vi "5. import Config.ini with include section.vi"() -> (3 "RS232_Device Config":T1={"Resource"="com5", "baud rate"=115200, "data bits"=8, "parity"=enum."Odd", "stop bits"=10})   [LabVIEW 2017]
doc: "## Referencing Configuration Files with [__include] (5. import Config.ini with include section.vi)\n\n### Overview\n\nThis example demonstrates CSM INI Variable Support API for referencing configuration files. You can use the reference configuration file feature to implement a distributed configuration file system.\n\n### Introduction\n\nIn configuration files loaded by CSM INI Variable Support API, if a [__include] section is present, the specified configuration files will be automatically referenced.\n\n**Notes:**\n\n- Relative paths are resolved relative to the current configuration file's path. Absolute paths are used directly.\n- Avoid circular dependencies, as they may lead to infinite loops. CSM INI Variable Support API maintains a record of loaded configuration files and skips loading if an attempt is made to load the same file a second time.\n- The key names in [__include] are not important. They serve only as identifiers. The paths in the values are what matters.\n- Configuration information in [__include] is loaded first, similar to loading first in a multi-file load scenario). Therefore, configuration items in the current configuration file will overwrite identical items in the referenced files.\n\n### Steps\n\n- Step1: Create multiple configuration files. Pay attention to internal reference relationships. Also note that [__include] is case-insensitive.\n- Step2: Load the file using `CSM - Load Configuration Variables From File.vi`.\n- Step3: Use `CSM - Configuration File Path.vi` to retrieve the paths of all currently loaded configuration files.\n- Step4: Attempt to read configuration information, noting the actual effective configuration after considering overwrite relationships."
uses:
  f65b758a-57a2-4ff6-b8fb-5289b55a65bc.vi
  f65b758a-57a2-4ff6-b8fb-5289b55a65bc.vi/99de0c97-112a-4c86-9094-c187659127e1.vi
  <userlib>/_NEVSTOP/Communicable State Machine(CSM)/Utility/Build Error Cluster.vi
  <vilib>/Utility/Data Type/Get Type Information.vi
  <userlib>/_NEVSTOP/Communicable State Machine(CSM)/addons/API-String-Arugments-Support/_Support/Data To SingleElementsArray_csm.vi
  <userlib>/_NEVSTOP/Communicable State Machine(CSM)/addons/API-String-Arugments-Support/_Support/Data To API String Arguments.vi
  INI-Static-Variable-Support/_Support/Parse Used Session and Name.vi
  INI-Static-Variable-Support/_Support/INI-FGV(lvlibp).vi
  INI-Static-Variable-Support/_Support/Populate String with INI Variable.vi
  <userlib>/_NEVSTOP/Communicable State Machine(CSM)/addons/API-String-Arugments-Support/_Support/Convert API String Arguments to Data(variant).vi
  <userlib>/_NEVSTOP/Communicable State Machine(CSM)/addons/API-String-Arugments-Support/_Support/SingleElementsArray To Data_csm.vi
  INI-Static-Variable-Support/INI-Static-Variable-Support.lvlib
panel:
  out "All Config Files":path[](array[path])
  # "#CSM-Example overview\n\nThis example demonstrates CSM INI Variable Support API for referencing configuration files. You can use the reference configuration file feature to implement a distributed configuration file system."
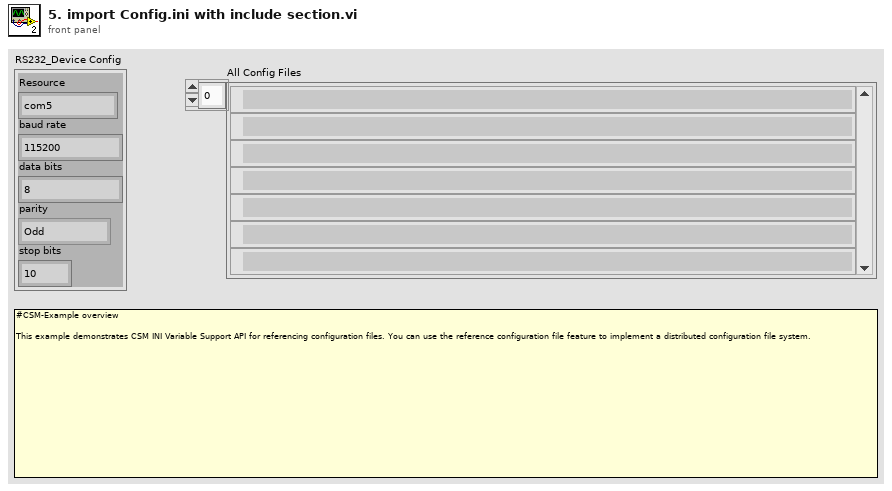
[diagram p1: front panel]
types:
  T1 = cluster{"Resource":string, "baud rate":u32, "data bits":u16, "parity":enum16{"None", "Odd", "Even", "Mark", "Space"}, "stop bits":u16}
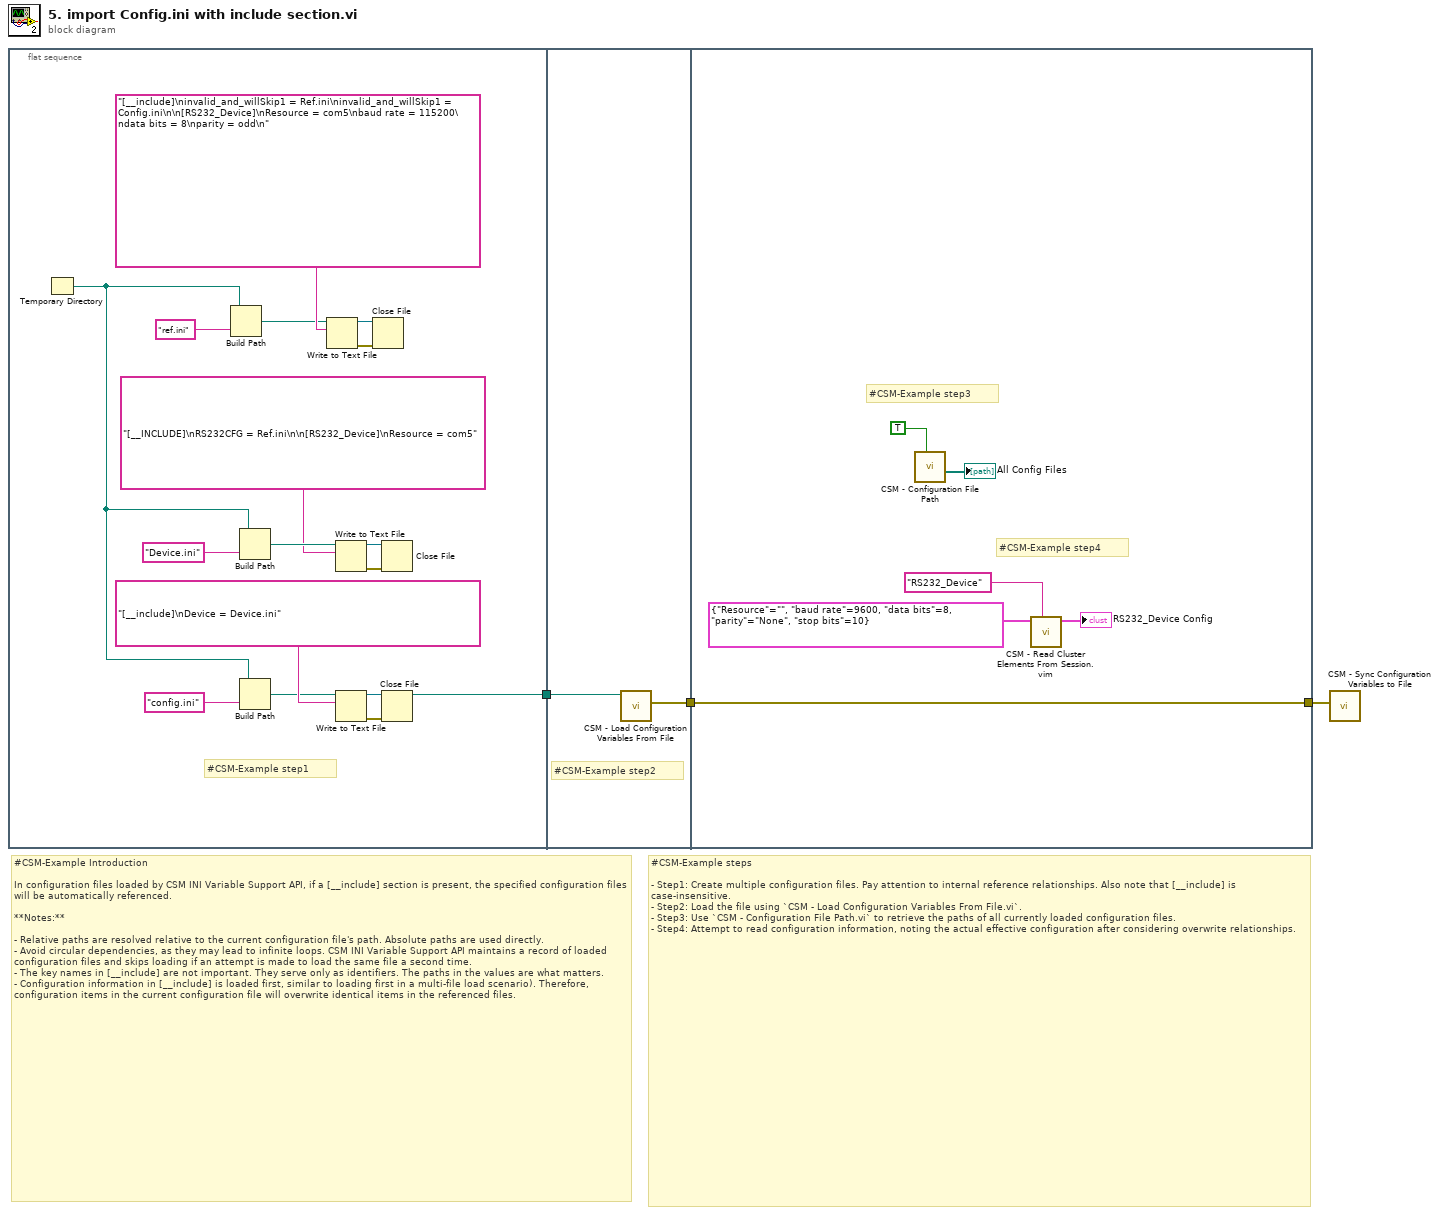
[diagram p0: block diagram]
diagram:
  # "#CSM-Example steps\n\n- Step1: Create multiple configuration files. Pay attention to internal reference relationships. Also note that [__include] is case-insensitive.\n- Step2: Load the file using `CSM - Load Configuration Variables From File.vi`.\n- Step3: Use `CSM - Configuration File Path.vi` to retrieve the paths of all currently loaded configuration files.\n- Step4: Attempt to read configuration information, noting the actual effective configuration after considering overwrite relationships."
  # "#CSM-Example Introduction\n\nIn configuration files loaded by CSM INI Variable Support API, if a [__include] section is present, the specified configuration files will be automatically referenced.\n\n**Notes:**\n\n- Relative paths are resolved relative to the current configuration file's path. Absolute paths are used directly.\n- Avoid circular dependencies, as they may lead to infinite loops. CSM INI Variable Support API maintains a record of loaded configuration files and skips loading if an attempt is made to load the same file a second time.\n- The key names in [__include] are not important. They serve only as identifiers. The paths in the values are what matters.\n- Configuration information in [__include] is loaded first, similar to loading first in a multi-file load scenario). Therefore, configuration items in the current configuration file will overwrite identical items in the referenced files."
  n1 = flat-sequence {
    tunnel: [w5] -> w1
    tunnel: [w22] -> w3
    tunnel: w1 -> [w21]
    tunnel: w3 -> [w23]
    tunnel: [w23] -> w2
    frame #0 {
      # "#CSM-Example step1"
      n2 = Temporary Directory() -> (w4:path)
      n3 = Build Path(base path=w4, name or relative path="ref.ini" ("Temporary File Extension (tmp)")) -> (appended path=w16:path)
      n4 = Build Path(base path=w4, name or relative path="Device.ini" ("Temporary File Extension (tmp)")) -> (appended path=w15:path)
      n5 = Build Path(base path=w4, name or relative path="config.ini" ("Temporary File Extension (tmp)")) -> (appended path=w6:path)
      n6 = Write to Text File(file (use dialog)=w16, text="[__include]\ninvalid_and_willSkip1 = Ref.ini\ninvalid_and_willSkip1 = Config.ini\n\n[RS232_Device]\nResource = com5\nbaud rate = 115200\ndata bits = 8\nparity = odd\n") -> (refnum out=w19:refnum<file>, error out=w20:errorcluster)  [unwired: 2 in, 1 out]
      n7 = Write to Text File(file (use dialog)=w15, text="[__INCLUDE]\nRS232CFG = Ref.ini\n\n[RS232_Device]\nResource = com5") -> (refnum out=w13:refnum<file>, error out=w12:errorcluster)  [unwired: 2 in, 1 out]
      n8 = Write to Text File(file (use dialog)=w6, text="[__include]\nDevice = Device.ini") -> (refnum out=w8:refnum<file>, error out=w9:errorcluster)  [unwired: 2 in, 1 out]
      n9 = Close File(refnum=w19, error in=w20) -> ()  [unwired: 2 out]
      n10 = Close File(refnum=w13, error in=w12) -> ()  [unwired: 2 out]
      n11 = Close File(refnum=w8, error in=w9) -> (path=w5:path)  [unwired: 1 out]
    }
    frame #1 {
      # "#CSM-Example step2"
      n12 = call "CSM - Load Configuration Variables From File.vi"("Configuration Path"=w21) -> ("error out"=w22:errorcluster)  [unwired: 8 in]
    }
    frame #2 {
      # "#CSM-Example step4"
      # "#CSM-Example step3"
      n13 = call "CSM - Configuration File Path.vi"("Include All Paths? (F)"=TRUE ("Include All Paths?(F)")) -> ("All Config Files"=→"All Config Files":path[])  [unwired: 6 in, 2 out]
      n14 = call "CSM - Read Cluster Elements From Session.vim"("Section Name (\"\" as Default)"="RS232_Device" ("Section Name(\"\" as Default)"), "Cluster"=T1 {"Resource"="", "baud rate"=9600, "data bits"=8, "parity"=enum."None", "stop bits"=10}) -> ("Cluster out"=→"RS232_Device Config":T1)  [unwired: 6 in, 1 out]
    }
  }
  n15 = call "CSM - Sync Configuration Variables to File.vi"("error in (no error)"=w2) -> ()  [unwired: 8 in, 1 out]
